vi "FdxCmdMonTrgWordIniCvi.vi"(8 "error in":errorcluster, 9 "MonTrgWordIni":T1, 11 "InstrumentHandle_port":u32) -> (0 "error out":errorcluster, 3 "InstrumentHandle_port":u32)   [LabVIEW 2020, in "AIM664LV.lvlib"]
doc: "This function initializes the Monitor Trigger Word. See Figure 8 which shows the dependencies and functionality of the trigger engine."
uses:
  AIM664LV.lvlib
  AFDX_LibraryAdmin/FdxGlobalDllPath.vi
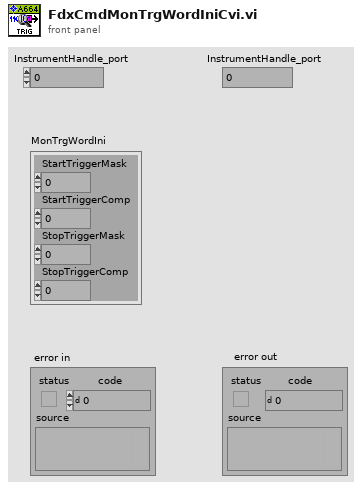
[diagram p1: front panel]
types:
  T1 = cluster{"StartTriggerMask":u32, "StartTriggerComp":u32, "StopTriggerMask":u32, "StopTriggerComp":u32}
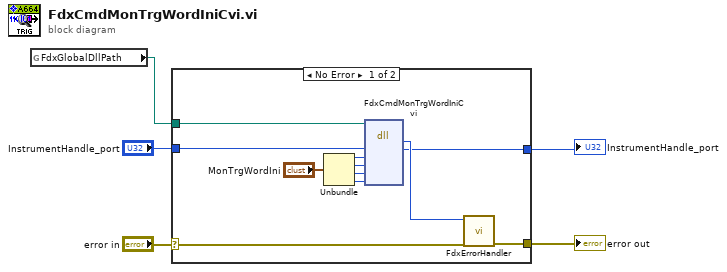
[diagram p0: block diagram]
diagram:
  n1 = global read "FdxGlobalDllPath.vi" "FdxGlobalDllPath"() -> (w3:path)
  n2 = case shown="No Error" "error in" {
    selector: "error in" -> [w15 w18]
    tunnel: [w16 w18] -> w5
    tunnel: w3 -> [w8 _]
    tunnel: [w7 w17] -> w2
    tunnel: "InstrumentHandle_port" -> [w6 w17]
    frame No Error {
      n3 = Unbundle("MonTrgWordIni") -> ("StartTriggerMask"=w12:u32, "StartTriggerComp"=w11:u32, "StopTriggerMask"=w10:u32, "StopTriggerComp"=w9:u32)
      n4 = dll-call lib="aim_fdx.19.dll" fn="FdxCmdMonTrgWordIniCvi"(path in=w8, "InstrumentHandle"=w6, "StartTriggerMask"=w12, "StartTriggerComp"=w11, "StopTriggerMask"=w10, "StopTriggerComp"=w9) -> ("status"=w14:i32, "InstrumentHandle"=w7:u32)  [unwired: 6 in, 2 out]
      n5 = call "FdxErrorHandler.vi"("error in"=w15, "AIM Error"=w14) -> ("error out"=w16:errorcluster)  [unwired: 9 in]
    }
    frame Error {
    }
  }
  "error out" <- w5
  "InstrumentHandle_port" <- w2
